vi "alloc_and_project_single_pattern_dmd.vi"(10 "pattern type":u16(ring) items=["from file", "all 0", "all 1"], 11 "File Path":path) -> (0 "return array":i32[](array[numeric]), 1 "SeqId":u32, 2 "DevId":u32, 3 "Image Out":T1)   [LabVIEW 2019]
uses:
  <vilib>/vision/Image Controls.llb/IMAQ Image.ctl
  <userlib>/alp4395/alp4395.lvlib
  <userlib>/alp4395/alp4395.dll
panel:
  out "function return 6":i32
  out "function return 9":i32
  out "function return 7":i32
  out "function return 5":i32
  out "function return 4":i32
  out "initialized array":u8[][][](array[numeric])
  out "array":u8[][][](array[numeric])
  out "function return 3":i32
  out "function return 2":i32
  out "function return 8":i32
  out "function return":i32
  in  "PictureTime":i32
  in  "PicNum":i32
  out "height":i32
  out "width":i32
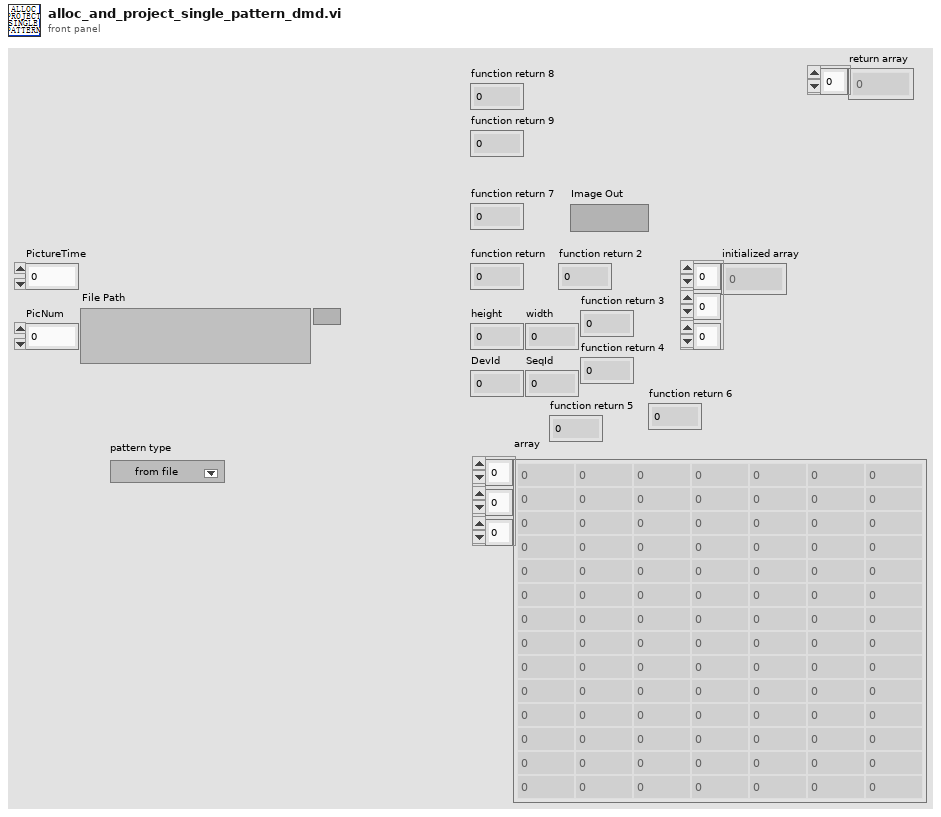
[diagram p1: front panel]
types:
  T1 = typedef "IMAQ Image.ctl" = refnum<image>
  T2 = typedef "Image Type" = u32
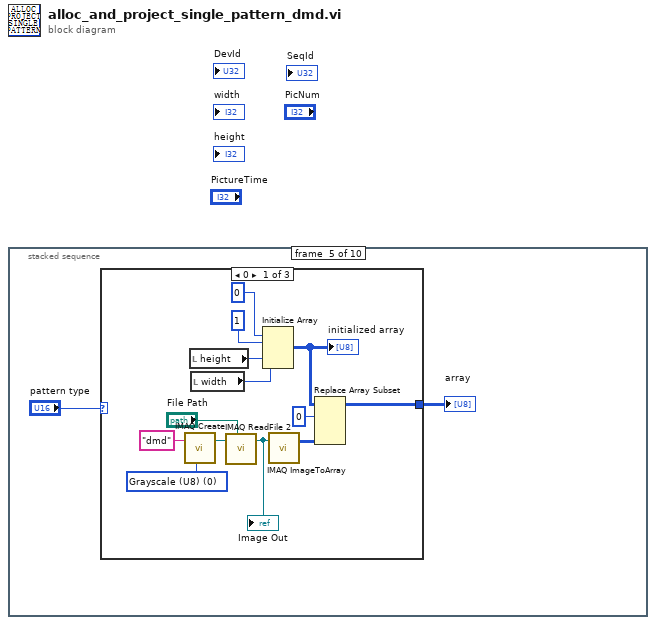
[diagram p0: block diagram]
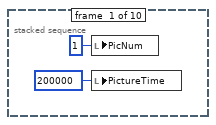
[diagram p2: hidden frame]
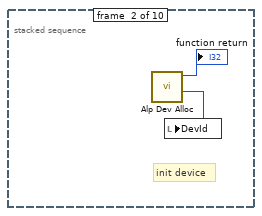
[diagram p3: hidden frame]
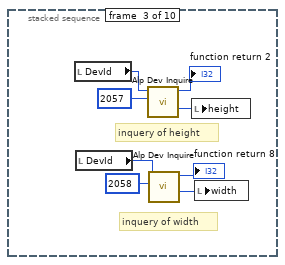
[diagram p4: hidden frame]
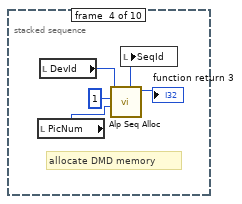
[diagram p5: hidden frame]
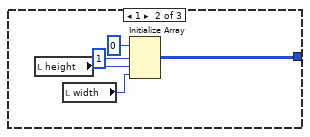
[diagram p6: hidden frame]
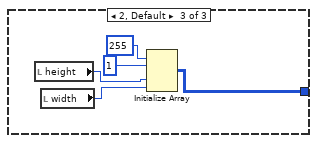
[diagram p7: hidden frame]
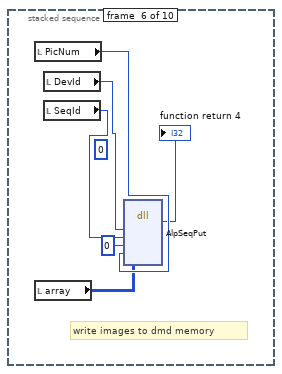
[diagram p8: hidden frame]
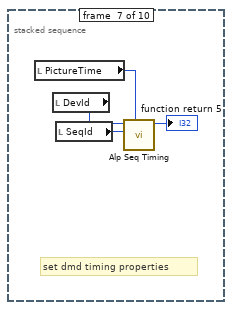
[diagram p9: hidden frame]
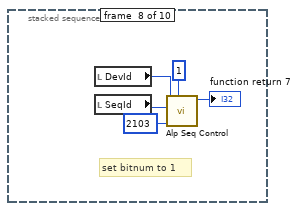
[diagram p10: hidden frame]
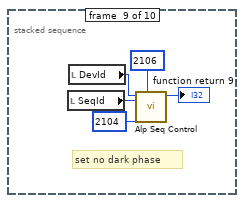
[diagram p11: hidden frame]
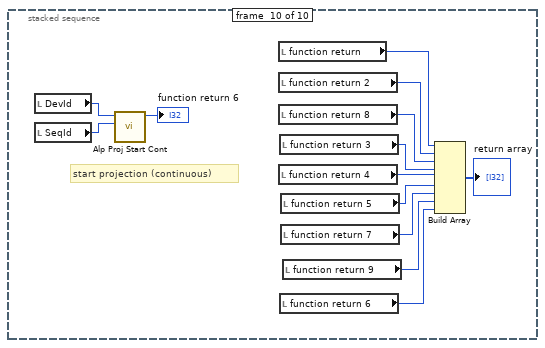
[diagram p12: hidden frame]
diagram:
  n1 = stacked-sequence {
    frame #0 {
      n2 = local write "PicNum"(1 ("PicNum")) -> ()
      n3 = local write "PictureTime"(200000 ("PictureTime")) -> ()
    }
    frame #1 {
      # "init device"
      n4 = call <userlib>:"Alp Dev Alloc.vi"() -> ("DeviceIdPtr out"=w4:u32, "function return"=→"function return":i32)  [unwired: 9 in, 1 out]
      n5 = local write "DevId"(w4) -> ()
    }
    frame #2 {
      # "inquery of width"
      # "inquery of height"
      n6 = local read "DevId"() -> (w10:u32)
      n7 = local read "DevId"() -> (w9:u32)
      n8 = call <userlib>:"Alp Dev Inquire.vi"("InquireType"=2057, "DeviceId"=w10) -> ("UserVarPtr out"=w11:i32, "function return"=→"function return 2":i32)  [unwired: 7 in, 1 out]
      n9 = call <userlib>:"Alp Dev Inquire.vi"("InquireType"=2058, "DeviceId"=w9) -> ("UserVarPtr out"=w7:i32, "function return"=→"function return 8":i32)  [unwired: 7 in, 1 out]
      n10 = local write "height"(w11) -> ()
      n11 = local write "width"(w7) -> ()
    }
    frame #3 {
      # "allocate DMD memory"
      n12 = local read "PicNum"() -> (w14:i32)
      n13 = local read "DevId"() -> (w17:u32)
      n14 = call <userlib>:"Alp Seq Alloc.vi"("PicNum"=w14, "BitPlanes"=1, "DeviceId"=w17) -> ("function return"=→"function return 3":i32, "SequenceIdPtr out"=w16:u32)  [unwired: 6 in, 1 out]
      n15 = local write "SeqId"(w16) -> ()
    }
    frame #4 {
      n16 = case shown="0" "pattern type" {
        tunnel: [w20 w33 w38] -> w18
        frame 0 {
          w23 = T2 0 items=["Grayscale (U8)", "Grayscale (I16)", "Grayscale (SGL)", "Complex (CSG)", "RGB (U32)", "HSL (U32)", "RGB (U64)", "Grayscale (U16)"] ("Image Type")
          n17 = call "IMAQ Create"("Image Name"="dmd", "Image Type"=w23) -> ("New Image"=w29:T1)  [unwired: 3 in, 1 out]
          n18 = local read "height"() -> (w22:i32)
          n19 = local read "width"() -> (w21:i32)
          n20 = call "IMAQ ReadFile 2"("File Path"="File Path", "Image"=w29) -> ("Image Out"=w28:T1)  [unwired: 5 in, 4 out]
          "Image Out" <- w28
          n21 = Initialize Array(u8 0 ("element"), 1 ("dimension size"), w22, w21) -> (w31:u8[][][])
          "initialized array" <- w31
          n22 = call "IMAQ ImageToArray"("Image"=w28) -> ("Image Pixels (U8)"=w30:u8[][])  [unwired: 3 in, 4 out]
          n23 = Replace Array Subset(array=w31, new element=w30, index (dim 0)=0 ("index (page)")) -> (w20:u8[][][])  [unwired: 2 in]
        }
        frame 1 {
          n24 = local read "height"() -> (w35:i32)
          n25 = local read "width"() -> (w34:i32)
          n26 = Initialize Array(u8 0 ("element"), 1 ("dimension size"), w35, w34) -> (w33:u8[][][])
        }
        frame 2, Default {
          n27 = local read "height"() -> (w40:i32)
          n28 = local read "width"() -> (w39:i32)
          n29 = Initialize Array(u8 255 ("element"), 1 ("dimension size"), w40, w39) -> (w38:u8[][][])
        }
      }
      "array" <- w18
    }
    frame #5 {
      (unwired) 0 ("PicOffset")
      # "write images to dmd memory"
      n30 = local read "PicNum"() -> (w46:i32)
      n31 = local read "array"() -> (w44:u8[][][])
      n32 = local read "DevId"() -> (w48:u32)
      n33 = local read "SeqId"() -> (w47:u32)
      n34 = dll-call lib="C:/Program Files/National Instruments/LabVIEW 2019/user.lib/alp4395/alp4395.dll" fn="AlpSeqPut"("DevID"=w48, "SeqID"=w47, "PicOffset"=0, "PicLoad"=w46, "UserArrayPtr"=w44) -> ("return type"=→"function return 4":i32)  [unwired: 3 in, 7 out]
    }
    frame #6 {
      # "set dmd timing properties"
      n35 = local read "PictureTime"() -> (w49:i32)
      n36 = local read "DevId"() -> (w52:u32)
      n37 = local read "SeqId"() -> (w51:u32)
      n38 = call <userlib>:"Alp Seq Timing.vi"("PictureTime"=w49, "SequenceId"=w51, "DeviceId"=w52) -> ("function return"=→"function return 5":i32)  [unwired: 7 in, 1 out]
    }
    frame #7 {
      # "set bitnum to 1"
      n39 = local read "DevId"() -> (w57:u32)
      n40 = local read "SeqId"() -> (w56:u32)
      n41 = call <userlib>:"Alp Seq Control.vi"("ControlValue"=1, "ControlType"=2103, "SequenceId"=w56, "DeviceId"=w57) -> ("function return"=→"function return 7":i32)  [unwired: 6 in, 1 out]
    }
    frame #8 {
      # "set no dark phase"
      n42 = local read "SeqId"() -> (w61:u32)
      n43 = local read "DevId"() -> (w62:u32)
      n44 = call <userlib>:"Alp Seq Control.vi"("ControlValue"=2106, "ControlType"=2104, "SequenceId"=w61, "DeviceId"=w62) -> ("function return"=→"function return 9":i32)  [unwired: 6 in, 1 out]
    }
    frame #9 {
      # "start projection (continuous)"
      n45 = local read "DevId"() -> (w75:u32)
      n46 = local read "SeqId"() -> (w74:u32)
      n47 = call <userlib>:"Alp Proj Start Cont.vi"("SequenceId"=w74, "DeviceId"=w75) -> ("function return"=→"function return 6":i32)  [unwired: 8 in, 1 out]
      n48 = local read "function return"() -> (w63:i32)
      n49 = local read "function return 2"() -> (w64:i32)
      n50 = local read "function return 8"() -> (w65:i32)
      n51 = local read "function return 4"() -> (w67:i32)
      n52 = local read "function return 3"() -> (w66:i32)
      n53 = local read "function return 6"() -> (w71:i32)
      n54 = local read "function return 5"() -> (w68:i32)
      n55 = local read "function return 7"() -> (w69:i32)
      n56 = local read "function return 9"() -> (w70:i32)
      n57 = Build Array(w63, w64, w65, w66, w67, w68, w69, w70, w71) -> (→"return array":i32[])
    }
  }
